vi "Update.vi"(8 "error in (no error)":errorcluster, 10 "Simulation Objects in":refnum<class "SimulationObject.lvclass">[](array[class]), 11 "PhysicsSystem in":refnum<class "PhysicsSystem.lvclass">) -> (0 "error out":errorcluster, 2 "Simulation Objects out":refnum<class "SimulationObject.lvclass">[](array[class]), 3 "PhysicsSystem out":refnum<class "PhysicsSystem.lvclass">)   [LabVIEW 2022 SP3, in "PhysicsSystem.lvclass"]
uses:
  PhysicsSystem.lvclass
  Objects/SimulationObject/SimulationObject.lvclass
  PhysicsSystem.lvclass/PhysicsSystem.ctl
  Math/Vector2/Vector2.lvclass
  Objects/Collisions/CollisionGrid/CollisionGrid.lvclass
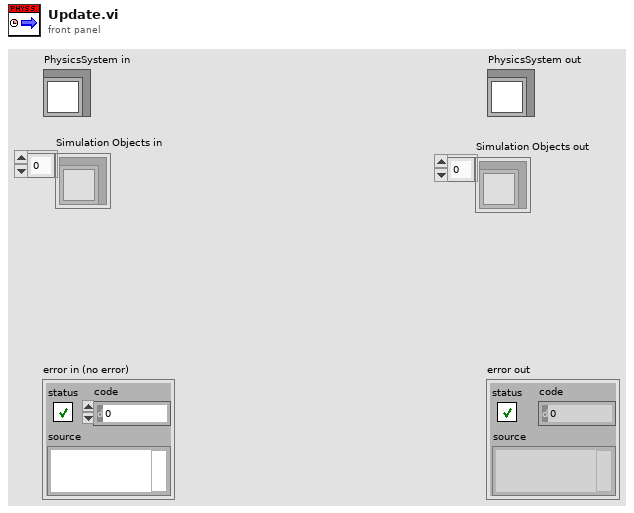
[diagram p1: front panel]
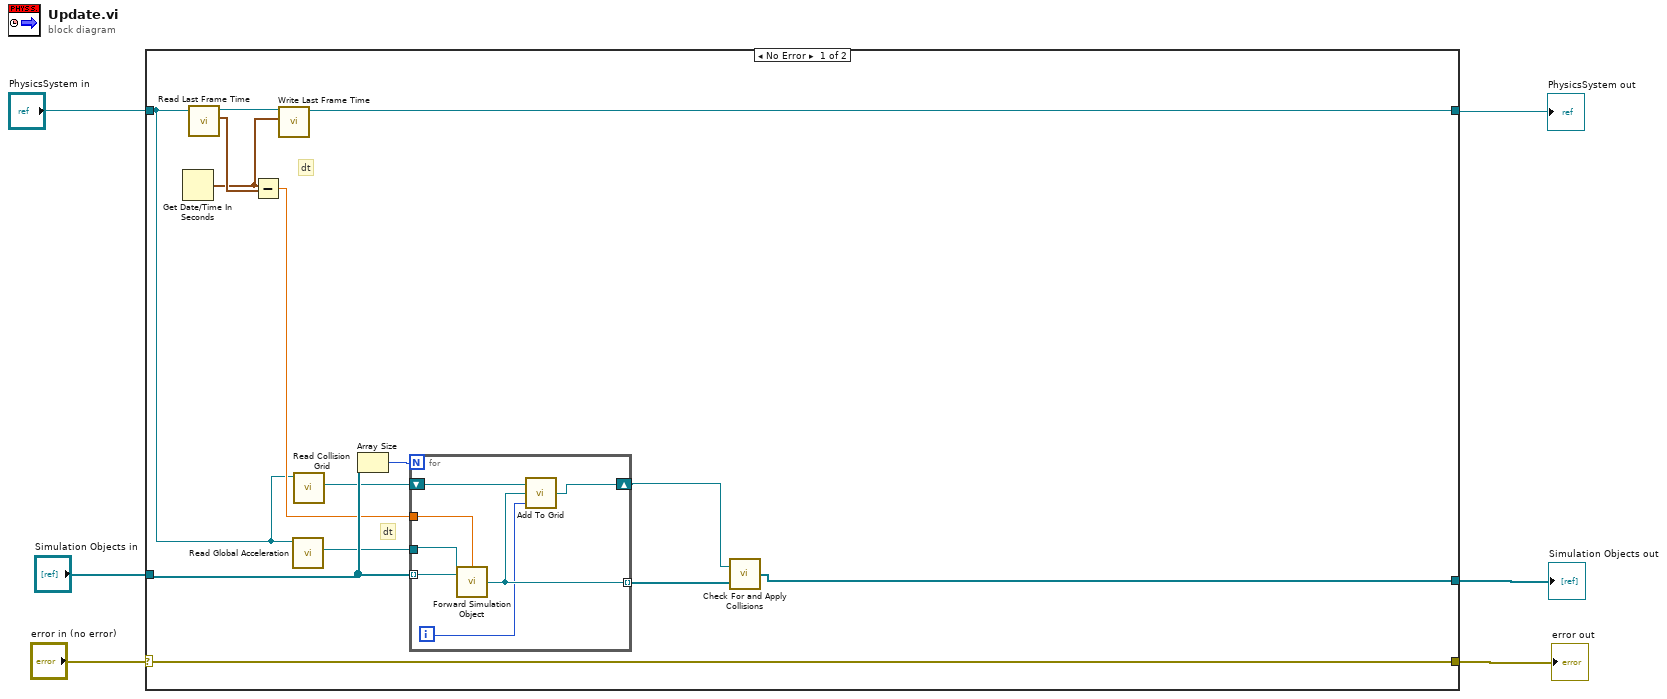
[diagram p0: block diagram]
diagram:
  n1 = case shown="No Error" "error in (no error)" {
    selector: "error in (no error)" -> [w20 w30]
    tunnel: [w20 w30] -> w5
    tunnel: [w16 w29] -> w4
    tunnel: "PhysicsSystem in" -> [w11 w29]
    tunnel: "Simulation Objects in" -> [w14 w28]
    tunnel: [w7 w28] -> w1
    frame No Error {
      # "dt"
      # "dt"
      n2 = Get Date/Time In Seconds() -> (seconds since 1Jan1904=w17:timestamp)
      n3 = call "Read Last Frame Time.vi"("PhysicsSystem in"=w11) -> ("Last Frame Time"=w18:timestamp, "PhysicsSystem out"=w19:refnum<class "PhysicsSystem.lvclass">)  [unwired: 8 in, 1 out]
      n4 = Subtract(x=w17, y=w18) -> (x-y=w12:dbl)
      n5 = call "Write Last Frame Time.vi"("Last Frame Time"=w17, "PhysicsSystem in"=w19) -> ("PhysicsSystem out"=w16:refnum<class "PhysicsSystem.lvclass">)  [unwired: 8 in, 1 out]
      n6 = call "Read Global Acceleration.vi"("PhysicsSystem in"=w11) -> ("Vector2.lvclass"=w13:refnum<class "Vector2.lvclass">)  [unwired: 8 in, 2 out]
      n7 = call "Read Collision Grid.vi"("PhysicsSystem in"=w11) -> ("Collision Grid out"=w10:refnum<class "CollisionGrid.lvclass">)  [unwired: 8 in, 2 out]
      n8 = Array Size(array=w14) -> (size(s)=w15:i32)
      n9 = for {
        N: w15 -> [_]
        tunnel: w14 -> [w27] mode=indexing
        tunnel: [w22] -> w9 mode=indexing
        tunnel: w13 -> [w26]
        tunnel: w12 -> [w25]
        shift-right: [w23] -> w8
        shift-left: w10 -> [w24]
        i -> [w21]
        n10 = call "Forward Simulation Object.vi"("Time step"=w25, "Global Acceleration in"=w26, "Simulation Object in"=w27) -> ("Simulation Object out"=w22:refnum<class "SimulationObject.lvclass">)
        n11 = call "Add To Grid.vi"("Object Index in"=w21, "Simulation Object in"=w22, "Collision Grid in"=w24) -> ("Collision Grid out"=w23:refnum<class "CollisionGrid.lvclass">)
      }
      n12 = call "Check For and Apply Collisions.vi"("Simulation Objects in"=w9, "Collision Grid"=w8) -> ("Simulation Objects out"=w7:refnum<class "SimulationObject.lvclass">[])
    }
    frame Error {
    }
  }
  "error out" <- w5
  "PhysicsSystem out" <- w4
  "Simulation Objects out" <- w1
